vi "Set google_protobuf_Field.vi"(7 "Complete Call (T)":bool=TRUE, 8 "error in (no error)":errorcluster, 10 "package_templatemessage":T1, 11 "gRPCid":T4) -> (0 "error out":errorcluster)   [LabVIEW 2020, in "FiveOhFeelsGood.lvlib"]
uses:
  FiveOhFeelsGood.lvlib
  <vilib>/gRPC/LabVIEW gRPC Library/Server API/typeDefs/grpcId.ctl
  google_protobuf_Field.ctl
  google_protobuf_Option.ctl
  google_protobuf_Any.ctl
  dcc74a39-081a-4bdd-860b-8ed792803c96.vi
  <vilib>/gRPC/LabVIEW gRPC Library/Server API/Server/Get Server DLL Path.vi
  <vilib>/Utility/error.llb/Error Cluster From Error Code.vi
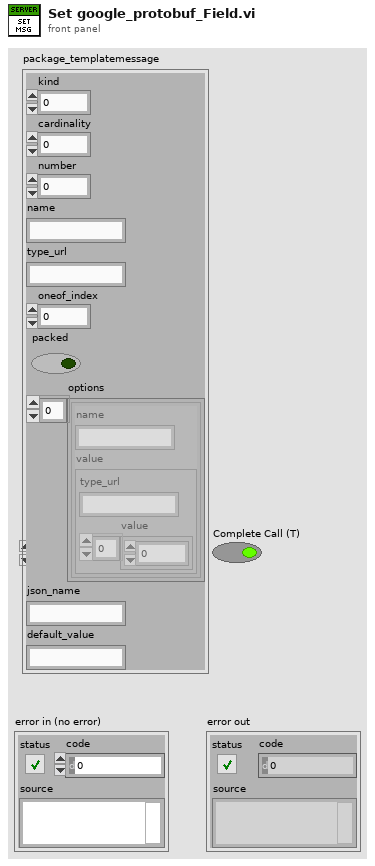
[diagram p1: front panel]
types:
  T1 = typedef "FiveOhFeelsGood.lvlib/google_protobuf_Field.ctl" = cluster{"kind":i32, "cardinality":i32, "number":i32, "name":string, "type_url":string, "oneof_index":i32, "packed":bool, "options":T2[], "json_name":string, "default_value":string}
  T2 = typedef "FiveOhFeelsGood.lvlib/google_protobuf_Option.ctl" = cluster{"name":string, "value":T3}
  T3 = typedef "FiveOhFeelsGood.lvlib/google_protobuf_Any.ctl" = cluster{"type_url":string, "value":u8[]}
  T4 = typedef "gprc-lvsupport-release.lvlib/grpcId.ctl" = u64
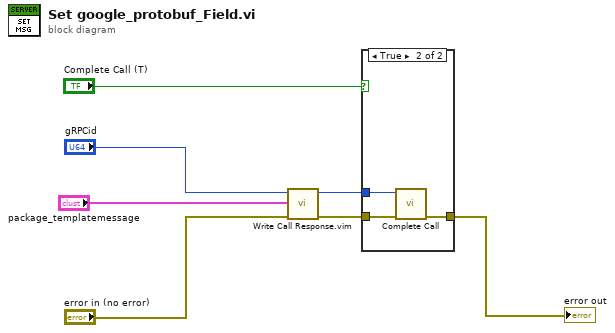
[diagram p0: block diagram]
diagram:
  n1 = call "Write Call Response.vim"("error in (no error)"="error in (no error)", "Response Data"="package_templatemessage", "gRPCid in"="gRPCid") -> ("error out"=w4:errorcluster, "gRPCid"=w5:T4)  [unwired: 7 in]
  n2 = case shown="True" "Complete Call (T)" {
    tunnel: [w8 w11] -> w7
    tunnel: w5 -> [_ w10]
    tunnel: w4 -> [w8 w9]
    frame False {
    }
    frame True {
      n3 = call <vilib>:"Complete Call.vi"("gRPCid"=w10, "error in (no error)"=w9) -> ("error out"=w11:errorcluster)  [unwired: 8 in]
    }
  }
  "error out" <- w7
